vi "Actor Core.vi"(8 "error in":errorcluster, 11 "Welcome in":refnum<class "Welcome.lvclass">) -> (0 "error out":errorcluster, 3 "Actor out":refnum<class "Actor.lvclass">)   [LabVIEW 2015, in "Item Actor.lvlib" / "Welcome.lvclass"]
doc: "(<B>Filename</B>: Actor Framework.lvlib:Actor.lvclass:Actor Core.vi)\n\nReceives messages to the actor, reacts to them, and initiates any error handling that may shut the actor down.\n\nDescendant classes may override this VI to append parallel tasks for the actor to complete while it handles messages. Overrides use the Call Parent Method node."
uses:
  Welcome.lvclass
  <vilib>/ActorFramework/Actor/Actor.lvclass
  <vilib>/ActorFramework/Actor/Actor.lvclass/Actor.ctl
  Store UI/StoreUI Messages/Display Item Msg/Display Item Msg.lvclass/Display Item Msg.ctl
  <vilib>/ActorFramework/Message Enqueuer/Message Enqueuer.lvclass/Message Enqueuer.ctl
  <vilib>/ActorFramework/Message Enqueuer/Enqueue.vi
  <vilib>/ActorFramework/Message Priority Queue/Priority Enqueue.vi
  Store UI/StoreUI Messages/Display Item Msg/Display Item Msg.lvclass
  Generic Item/Generic Item.lvclass
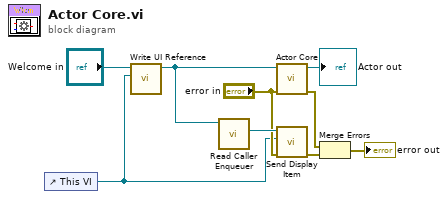
[diagram p0: block diagram]
diagram:
  n1 = control-ref of="This VI"() -> (w1:refnum<vi>)
  n2 = call "Write UI Reference.vi"("Item Panel"=w1, "Generic Item in"="Welcome in") -> ("Generic Item out"=w2:refnum<class "Welcome.lvclass">)  [unwired: 8 in, 1 out]
  n3 = call <vilib>:"Read Caller Enqueuer.vi"("Actor"=w2) -> ("Caller Enqueuer"=w8:refnum<class "Message Enqueuer.lvclass">)  [unwired: 10 in]
  n4 = call-parent "Actor Core.vi"("error in"="error in", "Generic Item in"=w2) -> ("error out"=w5:errorcluster, "Actor out"=→"Actor out":refnum<class "Actor.lvclass">)  [unwired: 8 in]
  n5 = call "Send Display Item.vi"("error in (no error)"="error in", "Item Panel"=w1, "Message Enqueuer"=w8) -> ("error out"=w6:errorcluster)  [unwired: 7 in, 1 out]
  n6 = Merge Errors(w5, w6) -> (→"error out":errorcluster)
